vi "Write Register (U32).vi"(0 "session in":refnum<k21>, 5 "device":refnum<k21>="$DefaultDevices", 7 "register address":u32 format="%.0x", 9 "data":u32 format="%.0x", 11 "error in (no error)":errorcluster) -> (4 "session out":refnum<k21>, 6 "device out":refnum<k21>, 8 "next register address":u32 format="%.0x", 15 "error out":errorcluster)   [LabVIEW 2020, in "SLSC.lvlib"]
doc: "Writes 32 bits of <B>data</B> to the <B>register address</B> of the specified <B>device</B>."
uses:
  <vilib>/SLSC/SLSC.lvlib
  nislsclvapi.dll
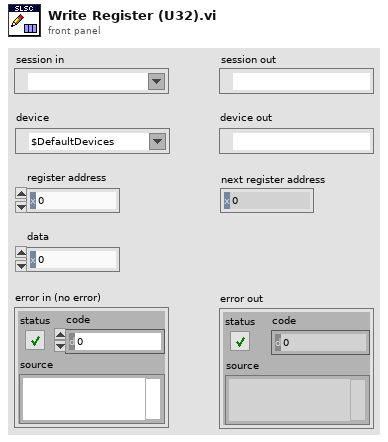
[diagram p1: front panel]
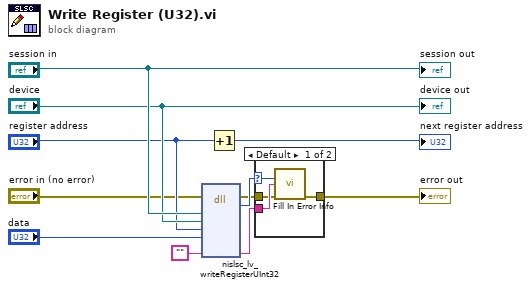
[diagram p0: block diagram]
diagram:
  n1 = dll-call lib="nislsclvapi.*" fn="nislsc_lv_writeRegisterUInt32"(error in="error in (no error)", "session"="session in", "deviceName"="device", "registerAddress"="register address", "data"="data", "extendedErrorInfo"="") -> (error out=w8:errorcluster, "return type"=w9:i32, "extendedErrorInfo"=w10:string)  [unwired: 8 in, 1 out]
  n2 = Increment(x="register address") -> (x+1=→"next register address":u32)
  n3 = case shown="Default" w9 {
    selector: w9 -> [w15 _]
    tunnel: w10 -> [w14 _]
    tunnel: w8 -> [w13 w16]
    tunnel: [w12 w16] -> w1
    frame Default {
      n4 = call <vilib>:"Fill In Error Info.vi"("status code"=w15, "extended error info"=w14, "error in"=w13) -> ("error out"=w12:errorcluster)  [unwired: 12 in]
    }
    frame 0 {
    }
  }
  "error out" <- w1
  "session out" <- "session in"
  "device out" <- "device"
